vi "Start.vi"(5 "Alias":string, 6 "Actor":refnum<class "Actor.lvclass">, 7 "Creator Attributes":refnum<class "Attributes.lvclass">, 9 "Queue of Self Attributes":refnum<queue>, 10 "Queue of Error":refnum<queue>) -> (0 "Error out":errorcluster)   [LabVIEW 2025, in "jettl.lvlib" / "Actor.lvlib"]
uses:
  Actor.lvlib
  Attributes/Attributes/Attributes.lvclass
  Actor/Actor.lvclass
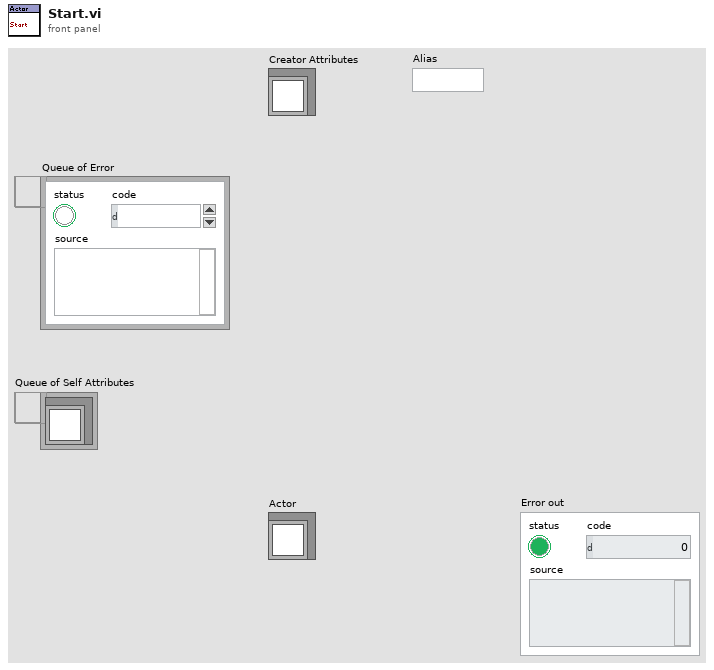
[diagram p1: front panel]
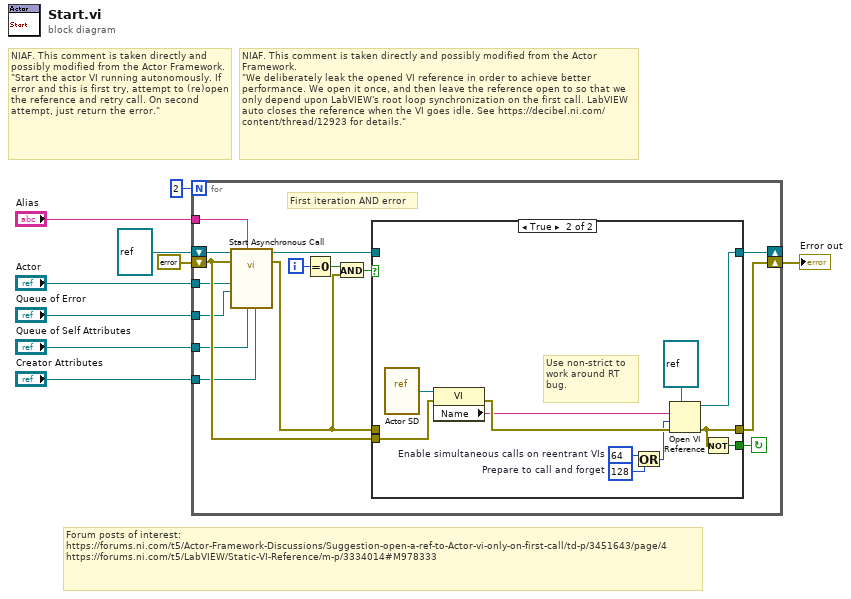
[diagram p0: block diagram]
diagram:
  # "Forum posts of interest:\nhttps://forums.ni.com/t5/Actor-Framework-Discussions/Suggestion-open-a-ref-to-Actor-vi-only-on-first-call/td-p/3451643/page/4\nhttps://forums.ni.com/t5/LabVIEW/Static-VI-Reference/m-p/3334014#M978333"
  # "NIAF. This comment is taken directly and possibly modified from the Actor Framework.\n\"We deliberately leak the opened VI reference in order to achieve better performance. We open it once, and then leave the reference open to so that we only depend upon LabVIEW's root loop synchronization on the first call. LabVIEW auto closes the reference when the VI goes idle. See https://decibel.ni.com/content/thread/12923 for details.\""
  # "NIAF. This comment is taken directly and possibly modified from the Actor Framework.\n\"Start the actor VI running autonomously. If error and this is first try, attempt to (re)open the reference and retry call. On second attempt, just return the error.\""
  n1 = for {
    N: 2 -> [_]
    shift-right: [w24] -> _
    shift-left: refnum<vi> refnum -> [w23]
    shift-right: [w21] -> w6
    shift-left: errorcluster {"status"=FALSE, "code"=0, "source"=""} ("error out") -> [w17]
    tunnel: "Queue of Error" -> [w16]
    tunnel: "Queue of Self Attributes" -> [w14]
    tunnel: "Creator Attributes" -> [w13]
    tunnel: "Alias" -> [w15]
    tunnel: "Actor" -> [w12]
    i -> [w19]
    stop <- w18 continue-if-true
    # "First iteration AND error"
    n2 = call-by-ref "Start Asynchronous Call"(reference=w23, error in=w17, "Creator Attributes"=w13, "Queue of Self Attributes"=w14, "Alias"=w15, "Queue of Error"=w16, "Actor in"=w12) -> (reference out=w22:refnum<vi>, error out=w10:errorcluster)  [unwired: 5 in, 2 out]
    n3 = Equal To 0?(x=w19) -> (x = 0?=w11:bool)
    n4 = And(x=w11, y=w10) -> (x .and. y?=w20:bool)
    n5 = case shown="True" w20 {
      tunnel: [w26 w35] -> w24
      tunnel: [w25 w33] -> w21
      tunnel: w22 -> [w26 _]
      tunnel: w10 -> [w25 _]
      tunnel: [_ w34] -> w18
      tunnel: w17 -> [_ w32]
      frame False {
      }
      frame True {
        w27 = 64  # Enable simultaneous calls on reentrant VIs
        w29 = 128  # Prepare to call and forget
        # "Use non-strict to work around RT bug."
        n6 = vi-ref "Actor SD.vi"() -> (w31:refnum<vi>)
        n7 = property class="VI"(reference=w31, error in=w32) -> (error out=w37:errorcluster, "Name"=w36:string)  [unwired: 1 out]
        n8 = Or(x=w27, y=w29) -> (x .or. y?=w28:i32)
        n9 = Open VI Reference(type specifier VI Refnum (for type only)=refnum<vi> refnum, vi path=w36, options=w28, error in (no error)=w37) -> (vi reference=w35:refnum<vi>, error out=w33:errorcluster)  [unwired: 2 in]
        n10 = Not(x=w33) -> (.not. x?=w34:bool)
      }
    }
  }
  "Error out" <- w6
